vi "Memory.Stats.vi"(8 "error in (no error)":errorcluster) -> (0 "error out":errorcluster, 3 "memory stats":T1 {"max allocated size" format="%.0x bytes"; "total allocated size" format="%.0x bytes"; "max free size" format="%.0x bytes"; "total free size" format="%.0x bytes"})   [LabVIEW 2016, in "Memory Manager.lvlib"]
doc: "Returns the current memory statistics for LabVIEW."
uses:
  Memory Manager.lvlib
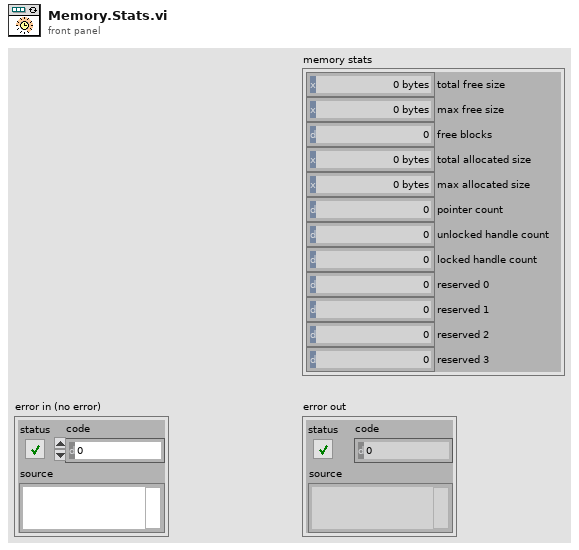
[diagram p1: front panel]
types:
  T1 = cluster{"total free size":i32, "max free size":i32, "free blocks":i32, "total allocated size":i32, "max allocated size":i32, "pointer count":i32, "unlocked handle count":i32, "locked handle count":i32, "reserved 0":i32, "reserved 1":i32, "reserved 2":i32, "reserved 3":i32}
  T2 = cluster{"total free size":i32, "max free size":i32, "number of free blocks":i32, "total allocated size":i32, "max allocated size":i32, "number of pointers":i32, "number of unlocked handles":i32, "number of locked handles":i32, "reserved 0":i32, "reserved 1":i32, "reserved 2":i32, "reserved 3":i32}
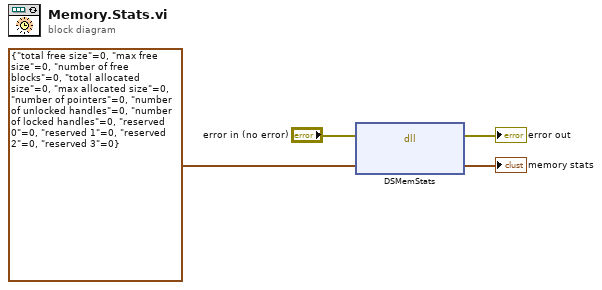
[diagram p0: block diagram]
diagram:
  n1 = dll-call lib="LabVIEW" fn="DSMemStats"(error in="error in (no error)", "MemStatRec"=T2 {"total free size"=0, "max free size"=0, "number of free blocks"=0, "total allocated size"=0, "max allocated size"=0, "number of pointers"=0, "number of unlocked handles"=0, "number of locked handles"=0, "reserved 0"=0, "reserved 1"=0, "reserved 2"=0, "reserved 3"=0}) -> (error out=→"error out":errorcluster, "MemStatRec"=→"memory stats":T2)  [unwired: 3 in, 1 out]
